vi "OSICS_Openport.vi"(8 "error in":errorcluster, 11 "VISA IN":refnum<visa-resource-name>) -> (0 "error out":errorcluster, 3 "VISA OUT":refnum<visa-resource-name>)   [LabVIEW 2014, in "OSICS_LIB.lvlib"]
doc: "This VI opens the data communication session."
uses:
  OSICS_LIB.lvlib
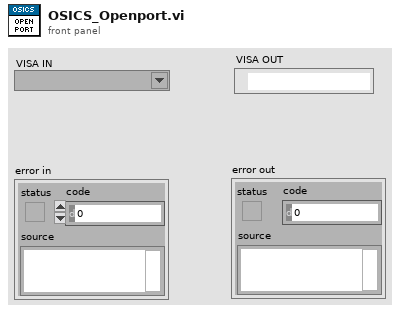
[diagram p1: front panel]
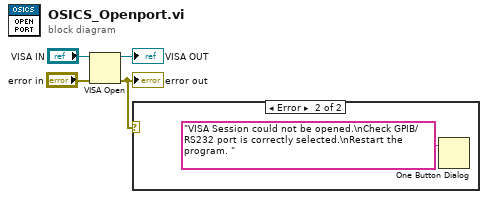
[diagram p0: block diagram]
diagram:
  n1 = VISA Open(error in (no error)="error in", VISA resource name="VISA IN") -> (VISA resource name=→"VISA OUT":refnum<visa-resource-name>, error out=w1:errorcluster)  [unwired: 3 in]
  "error out" <- w1
  n2 = case shown="Error" w1 {
    frame No Error {
    }
    frame Error {
      n3 = One Button Dialog(message="VISA Session could not be opened.\nCheck GPIB/RS232 port is correctly selected.\nRestart the program. ") -> ()  [unwired: 1 in, 1 out]
    }
  }
